vi "CreateNewCaseStructure.vi"(11 "FrameNames":string[](array[string])) -> ()   [LabVIEW 2015]
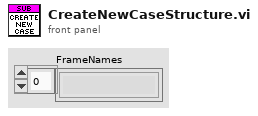
[diagram p1: front panel]
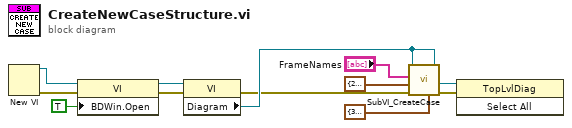
[diagram p0: block diagram]
diagram:
  n1 = New VI() -> (0:w9:errorcluster, 3:w8:refnum<vi>)  [unwired: 7 in]
  n2 = property class="VI"(reference=w8, error in=w9, "BDWin.Open"=TRUE ("Block Diagram Window:Open")) -> (reference out=w11:refnum<vi>, error out=w7:errorcluster)
  n3 = property class="VI"(reference=w11, error in=w7) -> (error out=w1:errorcluster, "Diagram"=w2:refnum<vi>)  [unwired: 1 out]
  n4 = call "SubVI_CreateCase.vi"("Bounds"=cluster{"Width":u32, "Height":u32} {"Width"=360, "Height"=240}, "error in (no error)"=w1, "Point"=cluster{"Horizontal":i16, "Vertical":i16} {"Horizontal"=240, "Vertical"=160}, "FrameNames"="FrameNames", "Diagram in"=w2) -> ("error out"=w5:errorcluster)  [unwired: 4 in, 2 out]
  n5 = invoke class="TopLvlDiag" method="Select All"(reference=w2, error in=w5) -> ()  [unwired: 1 in, 3 out]
